vi "Init_Read_INI_file.vi"(0 "Path to INI":string="C:\\ProgramData\\Noffz\\mmW_Service\\mmW_Service.ini", 11 "error in (no error)":errorcluster) -> (15 "error out":errorcluster)   [LabVIEW 2019, in "Service.lvlib"]
uses:
  Service.lvlib
  TypeDef/AppData.ctl
  MsgQ/TypeDefs/CommandsQ.ctl
  MsgQ/TypeDefs/MsgQ_Commands.ctl
  <vilib>/Utility/config.llb/Read Key (String).vi
  <vilib>/Utility/config.llb/Read Key (Double).vi
  <vilib>/Utility/config.llb/NI_LVConfig.lvlib
  MsgQ/MsgQ.lvlib
panel:
  out "section names":string[](array[string])
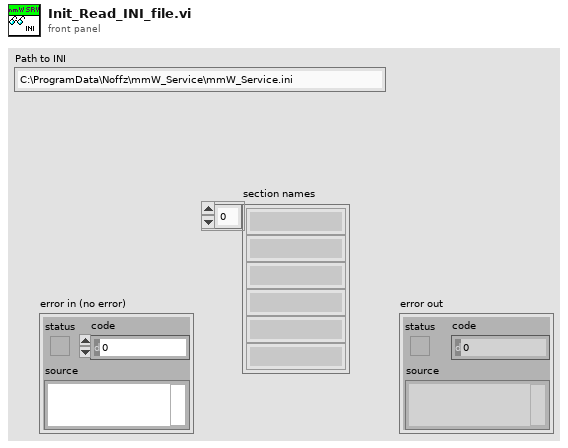
[diagram p1: front panel]
types:
  T1 = typedef "NI_LVConfig.lvlib/Config Data RefNum.ctl" = refnum<k1>
  T2 = typedef "Service.lvlib/AppData.ctl" = cluster{"MsgQ":refnum<queue>, "Stop?":bool, "zmq sessions":cluster{"Control_endpoint":string, "Instr_endpoint":string}, "control-loop":cluster{"fromUI-Q":refnum<queue>, "toUI":refnum<user-event>, "Control_endpoint":string}, "UI-loop":cluster{"evnt_ref":refnum<event-registration>}, "logging":cluster{"level":dbl, "verbosity":dbl, "path":string, "Listener_ID":string}, "general_settings":cluster{"mmW_instr_ini_path":string, "mmW_instr_pid_path":string}}
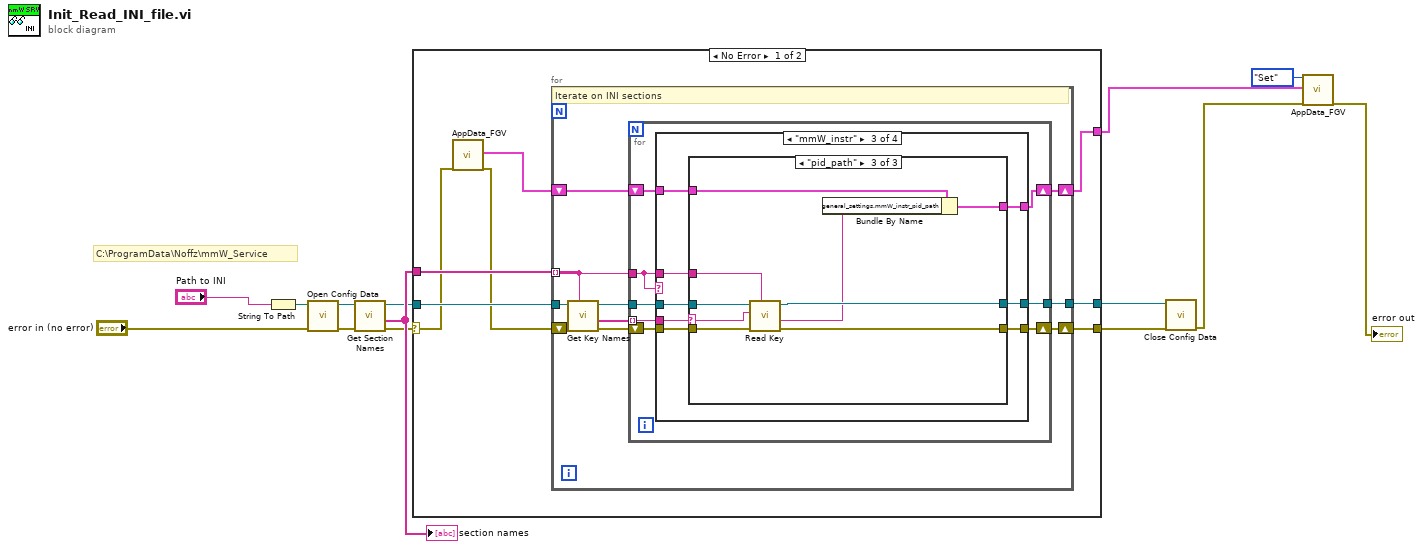
[diagram p0: block diagram]
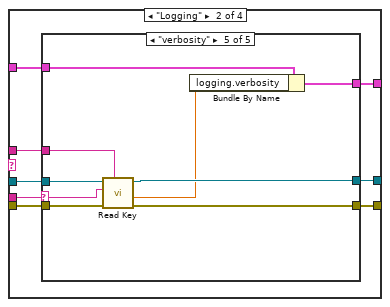
[diagram p3: hidden frame]
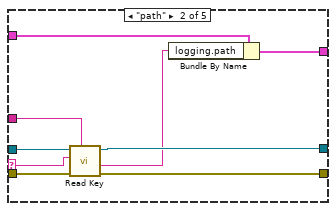
[diagram p5: hidden frame]
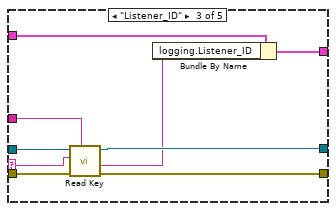
[diagram p6: hidden frame]
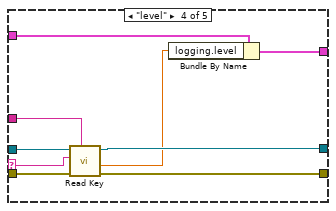
[diagram p7: hidden frame]
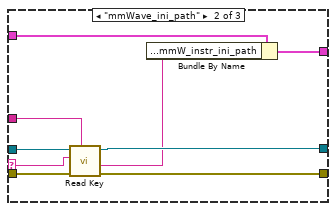
[diagram p9: hidden frame]
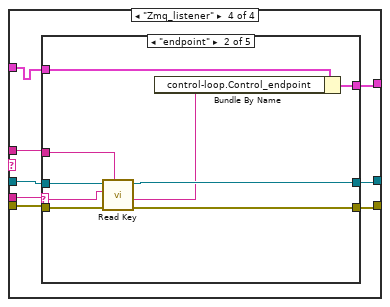
[diagram p10: hidden frame]
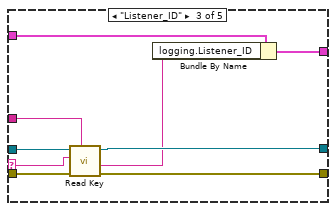
[diagram p12: hidden frame]
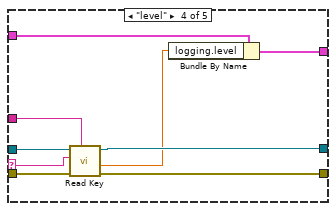
[diagram p13: hidden frame]
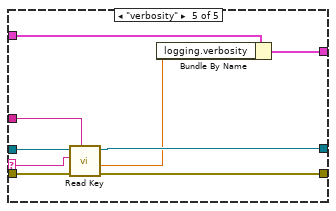
[diagram p14: hidden frame]
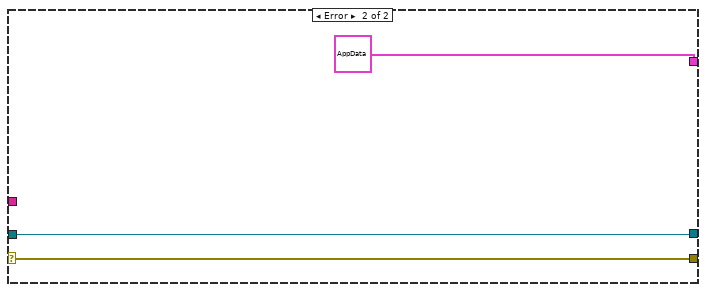
[diagram p15: hidden frame]
diagram:
  # "C:\\ProgramData\\Noffz\\mmW_Service"
  n1 = String To Path(string="Path to INI") -> (path=w11:path)
  n2 = call <vilib>:"Open Config Data.vi"("error in (no error)"="error in (no error)", "configuration file path"=w11) -> ("error out"=w13:errorcluster, "refnum"=w14:T1)  [unwired: 7 in, 1 out]
  n3 = call <vilib>:"Get Section Names.vi"("error in (no error)"=w13, "refnum"=w14) -> ("error out"=w8:errorcluster, "section names"=w10:string[], "refnum out"=w9:T1)  [unwired: 7 in]
  "section names" <- w10
  n4 = case shown="No Error" w8 {
    selector: w8 -> [w16 w168]
    tunnel: w10 -> [w22 _]
    tunnel: w9 -> [w21 w169]
    tunnel: [w20 w169] -> w7
    tunnel: [w19 w168] -> w6
    tunnel: [w18 T2 {"MsgQ"=refnum, "Stop?"=FALSE, "zmq sessions"={"Control_endpoint"="", "Instr_endpoint"=""}, "control-loop"={"fromUI-Q"=refnum, "toUI"=refnum, "Control_endpoint"=""}, "UI-loop"={"evnt_ref"=refnum}, "logging"={"level"=0.0, "verbosity"=0.0, "path"="", "Listener_ID"=""}, "general_settings"={"mmW_instr_ini_path"="", "mmW_instr_pid_path"=""}} ("AppData out")] -> w5
    frame No Error {
      n5 = call "AppData_FGV.vi"("error in (no error)"=w16) -> ("AppData out"=w17:T2, "error out"=w15:errorcluster)  [unwired: 17 in]
      n6 = for {
        tunnel: w22 -> [w25] mode=indexing
        tunnel: w21 -> [w31]
        tunnel: [w27] -> w20
        shift-right: [w26] -> w19
        shift-left: w15 -> [w32]
        shift-right: [w23] -> w18
        shift-left: w17 -> [w24]
        # "Iterate on INI sections"
        n7 = call <vilib>:"Get Key Names.vi"("section"=w25, "error in (no error)"=w32, "refnum"=w31) -> ("error out"=w30:errorcluster, "key names"=w28:string[], "refnum out"=w29:T1)  [unwired: 5 in, 1 out]
        n8 = for {
          tunnel: w28 -> [w38] mode=indexing
          tunnel: w29 -> [w40]
          tunnel: [w37] -> w27
          shift-right: [w36] -> w26
          shift-left: w30 -> [w39]
          tunnel: w25 -> [w35]
          shift-right: [w33] -> w23
          shift-left: w24 -> [w34]
          n9 = case shown="\"mmW_instr\"" w35 {
            tunnel: w40 -> [w43 w51 w98 w124]
            tunnel: w39 -> [w41 w50 w97 w122]
            tunnel: w38 -> [_ w46 w93 w123]
            tunnel: [w43 w49 w96 w120] -> w37
            tunnel: [w41 w48 w95 w121] -> w36
            tunnel: w35 -> [_ w47 w94 w125]
            tunnel: w34 -> [w42 w45 w92 w127]
            tunnel: [w42 w44 w91 w126] -> w33
            frame "False", Default {
            }
            frame "Logging" {
              n10 = case shown="\"verbosity\"" w46 {
                selector: w46 -> [_ w58 w67 w76 w85]
                tunnel: w51 -> [w54 w63 w72 w81 w90]
                tunnel: w50 -> [w52 w62 w71 w80 w89]
                tunnel: [w54 w61 w70 w79 w88] -> w49
                tunnel: [w52 w60 w69 w78 w87] -> w48
                tunnel: w47 -> [_ w59 w68 w77 w86]
                tunnel: w45 -> [w53 w57 w66 w75 w84]
                tunnel: [w53 w55 w64 w73 w82] -> w44
                frame "False", Default {
                }
                frame "path" {
                  n11 = call-poly <vilib>:"Read Key.vi"("section"=w59, "error in (no error)"=w62, "key"=w58, "refnum"=w63) -> ("error out"=w60:errorcluster, "value"=w56:string, "refnum out"=w61:T1)  [unwired: 4 in, 1 out]
                  n12 = Bundle By Name(cluster=w57, "logging.path"=w56) -> (w55:T2)
                }
                frame "Listener_ID" {
                  n13 = call-poly <vilib>:"Read Key.vi"("section"=w68, "error in (no error)"=w71, "key"=w67, "refnum"=w72) -> ("error out"=w69:errorcluster, "value"=w65:string, "refnum out"=w70:T1)  [unwired: 4 in, 1 out]
                  n14 = Bundle By Name(cluster=w66, "logging.Listener_ID"=w65) -> (w64:T2)
                }
                frame "level" {
                  n15 = call-poly <vilib>:"Read Key.vi"("section"=w77, "error in (no error)"=w80, "key"=w76, "refnum"=w81) -> ("error out"=w78:errorcluster, "value"=w74:dbl, "refnum out"=w79:T1)  [unwired: 4 in, 1 out]
                  n16 = Bundle By Name(cluster=w75, "logging.level"=w74) -> (w73:T2)
                }
                frame "verbosity" {
                  n17 = call-poly <vilib>:"Read Key.vi"("section"=w86, "error in (no error)"=w89, "key"=w85, "refnum"=w90) -> ("error out"=w87:errorcluster, "value"=w83:dbl, "refnum out"=w88:T1)  [unwired: 4 in, 1 out]
                  n18 = Bundle By Name(cluster=w84, "logging.verbosity"=w83) -> (w82:T2)
                }
              }
            }
            frame "mmW_instr" {
              n19 = case shown="\"pid_path\"" w93 {
                selector: w93 -> [_ w105 w114]
                tunnel: w98 -> [w101 w110 w119]
                tunnel: w97 -> [w99 w109 w118]
                tunnel: [w101 w108 w117] -> w96
                tunnel: [w99 w107 w116] -> w95
                tunnel: w94 -> [_ w106 w115]
                tunnel: w92 -> [w100 w104 w113]
                tunnel: [w100 w102 w111] -> w91
                frame "False", Default {
                }
                frame "mmWave_ini_path" {
                  n20 = call-poly <vilib>:"Read Key.vi"("section"=w106, "error in (no error)"=w109, "key"=w105, "refnum"=w110) -> ("error out"=w107:errorcluster, "value"=w103:string, "refnum out"=w108:T1)  [unwired: 4 in, 1 out]
                  n21 = Bundle By Name(cluster=w104, "general_settings.mmW_instr_ini_path"=w103) -> (w102:T2)
                }
                frame "pid_path" {
                  n22 = call-poly <vilib>:"Read Key.vi"("section"=w115, "error in (no error)"=w118, "key"=w114, "refnum"=w119) -> ("error out"=w116:errorcluster, "value"=w112:string, "refnum out"=w117:T1)  [unwired: 4 in, 1 out]
                  n23 = Bundle By Name(cluster=w113, "general_settings.mmW_instr_pid_path"=w112) -> (w111:T2)
                }
              }
            }
            frame "Zmq_listener" {
              n24 = case shown="\"endpoint\"" w123 {
                selector: w123 -> [_ w134 w143 w152 w161]
                tunnel: w124 -> [w130 w139 w148 w157 w166]
                tunnel: w122 -> [w128 w138 w147 w156 w165]
                tunnel: [w130 w137 w146 w155 w164] -> w120
                tunnel: [w128 w136 w145 w154 w163] -> w121
                tunnel: w125 -> [_ w135 w144 w153 w162]
                tunnel: w127 -> [w129 w133 w142 w151 w160]
                tunnel: [w129 w131 w140 w149 w158] -> w126
                frame "False", Default {
                }
                frame "endpoint" {
                  n25 = call-poly <vilib>:"Read Key.vi"("section"=w135, "error in (no error)"=w138, "key"=w134, "refnum"=w139) -> ("error out"=w136:errorcluster, "value"=w132:string, "refnum out"=w137:T1)  [unwired: 4 in, 1 out]
                  n26 = Bundle By Name(cluster=w133, "control-loop.Control_endpoint"=w132) -> (w131:T2)
                }
                frame "Listener_ID" {
                  n27 = call-poly <vilib>:"Read Key.vi"("section"=w144, "error in (no error)"=w147, "key"=w143, "refnum"=w148) -> ("error out"=w145:errorcluster, "value"=w141:string, "refnum out"=w146:T1)  [unwired: 4 in, 1 out]
                  n28 = Bundle By Name(cluster=w142, "logging.Listener_ID"=w141) -> (w140:T2)
                }
                frame "level" {
                  n29 = call-poly <vilib>:"Read Key.vi"("section"=w153, "error in (no error)"=w156, "key"=w152, "refnum"=w157) -> ("error out"=w154:errorcluster, "value"=w150:dbl, "refnum out"=w155:T1)  [unwired: 4 in, 1 out]
                  n30 = Bundle By Name(cluster=w151, "logging.level"=w150) -> (w149:T2)
                }
                frame "verbosity" {
                  n31 = call-poly <vilib>:"Read Key.vi"("section"=w162, "error in (no error)"=w165, "key"=w161, "refnum"=w166) -> ("error out"=w163:errorcluster, "value"=w159:dbl, "refnum out"=w164:T1)  [unwired: 4 in, 1 out]
                  n32 = Bundle By Name(cluster=w160, "logging.verbosity"=w159) -> (w158:T2)
                }
              }
            }
          }
        }
      }
    }
    frame Error {
    }
  }
  n33 = call <vilib>:"Close Config Data.vi"("error in (no error)"=w6, "refnum"=w7) -> ("error out"=w2:errorcluster)  [unwired: 8 in, 1 out]
  n34 = call "AppData_FGV.vi"("Mode"=enum16{"Get", "Set", "Reset"}."Set", "AppData in"=w5, "error in (no error)"=w2) -> ("error out"=→"error out":errorcluster)  [unwired: 15 in, 1 out]
